vi "Process_single.vi"(0 "Arrays in":T2, 1 "output cluster":cluster{dbl, dbl, dbl, dbl}, 2 "Magnetic field":dbl, 3 "Calibration Constant (1/deg)":dbl) -> (5 "Magnetic_field_array":dbl[](array[numeric]), 6 "Time":dbl, 7 "Lockin_Y_array (V)":dbl[](array[numeric]), 8 "Time array (s)":dbl[](array[numeric]), 9 "Moke out":T1, 10 "LockIn Y":dbl, 11 "Lockin_R_array (V)":dbl[](array[numeric]), 12 "Lockin_Theta_array":dbl[](array[numeric]), 13 "LockIn R":dbl, 14 "LockIn X":dbl, 15 "MOKE_array (deg)":dbl[](array[numeric]), 16 "Lockin_X_array (V)":dbl[](array[numeric]), 17 "LockIn Theta":dbl, 18 "Dc_Voltage_array (V)":dbl[](array[numeric]))   [LabVIEW 2015]
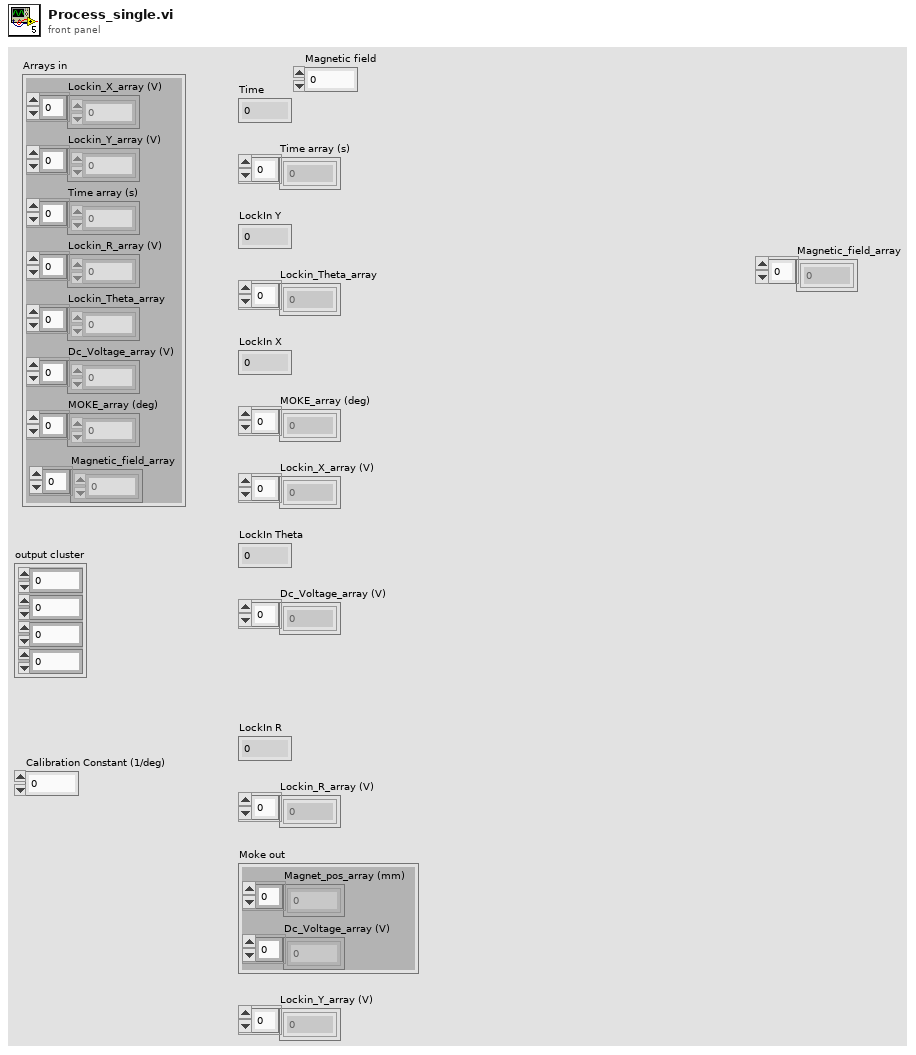
[diagram p1: front panel]
types:
  T1 = cluster{"Magnet_pos_array (mm)":dbl[], "Dc_Voltage_array (V)":dbl[]}
  T2 = cluster{"Lockin_X_array (V)":dbl[], "Lockin_Y_array (V)":dbl[], "Time array (s)":dbl[], "Lockin_R_array (V)":dbl[], "Lockin_Theta_array":dbl[], "Dc_Voltage_array (V)":dbl[], "MOKE_array (deg)":dbl[], "Magnetic_field_array":dbl[]}
  T3 = cluster{"Magnetic_field_array":dbl[], "Lockin_R_array (V)":dbl[]}
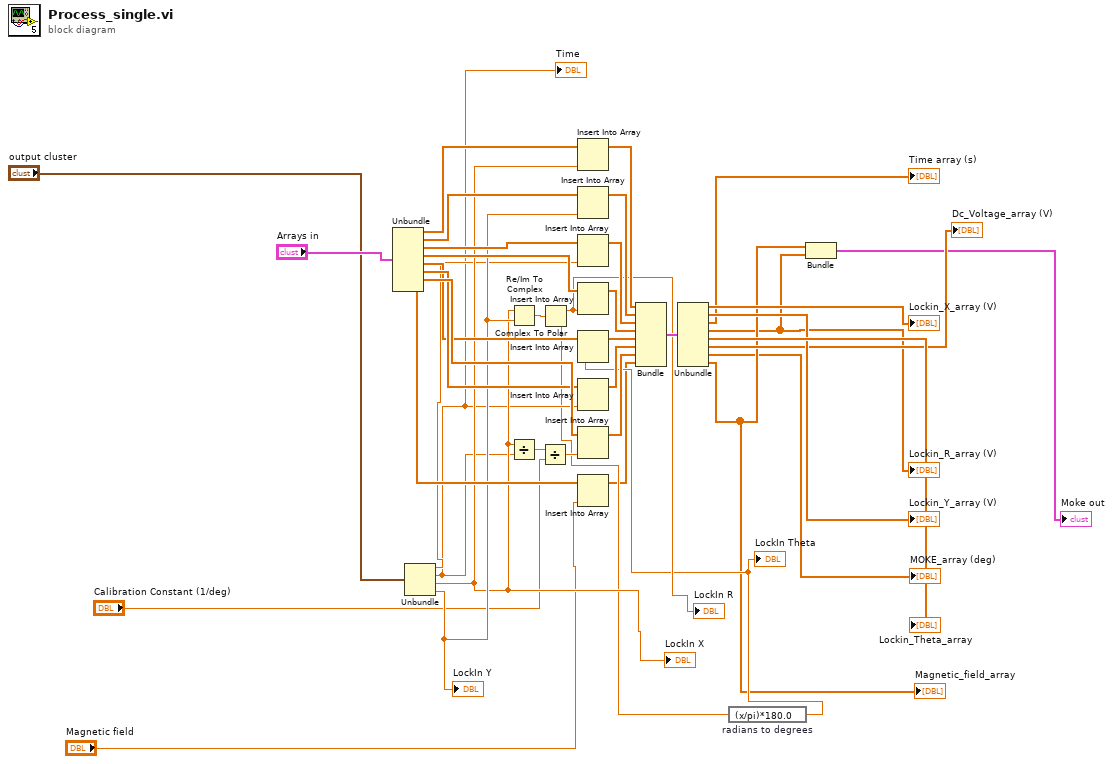
[diagram p0: block diagram]
diagram:
  n1 = Unbundle("Arrays in") -> ("Lockin_X_array (V)"=w22:dbl[], "Lockin_Y_array (V)"=w23:dbl[], "Time array (s)"=w24:dbl[], "Lockin_R_array (V)"=w25:dbl[], "Lockin_Theta_array"=w26:dbl[], "Dc_Voltage_array (V)"=w27:dbl[], "MOKE_array (deg)"=w28:dbl[], "Magnetic_field_array"=w29:dbl[])
  n2 = Unbundle("output cluster") -> (w16:dbl, w15:dbl, w17:dbl, w18:dbl)
  "LockIn Y" <- w18
  "LockIn X" <- w17
  "Time" <- w15
  n3 = Re/Im To Complex(1:w18, 2:w17) -> (0:w19:cdb)
  n4 = Divide(x=w17, y=w15) -> (x/y=w11:dbl)
  n5 = Divide(x=w11, y="Calibration Constant (1/deg)") -> (x/y=w13:dbl)
  n6 = Complex To Polar(r * e^(i*theta)=w19) -> (r=w20:dbl, theta=w10:dbl)
  "LockIn R" <- w20
  n7 = Insert Into Array(array=w22, new element=w17) -> (w32:dbl[])  [unwired: 1 in]
  n8 = Insert Into Array(array=w23, new element=w18) -> (w34:dbl[])  [unwired: 1 in]
  n9 = Insert Into Array(array=w24, new element=w16) -> (w31:dbl[])  [unwired: 1 in]
  n10 = Insert Into Array(array=w25, new element=w20) -> (w36:dbl[])  [unwired: 1 in]
  n11 = Insert Into Array(array=w27, new element=w15) -> (w39:dbl[])  [unwired: 1 in]
  n12 = Insert Into Array(array=w28, new element=w13) -> (w40:dbl[])  [unwired: 1 in]
  n13 = Insert Into Array(array=w29, new element="Magnetic field") -> (w6:dbl[])  [unwired: 1 in]
  n14 = expression code="(x/pi)*180.0" "radians to degrees"(w10) -> (w7:dbl)
  "LockIn Theta" <- w7
  n15 = Insert Into Array(array=w26, new element=w7) -> (w37:dbl[])  [unwired: 1 in]
  n16 = Bundle("Lockin_X_array (V)"=w32, "Lockin_Y_array (V)"=w34, "Time array (s)"=w31, "Lockin_R_array (V)"=w36, "Lockin_Theta_array"=w37, "Dc_Voltage_array (V)"=w39, "MOKE_array (deg)"=w40, "Magnetic_field_array"=w6) -> (w30:T2)  [unwired: 1 in]
  n17 = Unbundle(w30) -> ("Lockin_X_array (V)"=→"Lockin_X_array (V)":dbl[], "Lockin_Y_array (V)"=→"Lockin_Y_array (V)":dbl[], "Time array (s)"=→"Time array (s)":dbl[], "Lockin_R_array (V)"=w1:dbl[], "Lockin_Theta_array"=→"Lockin_Theta_array":dbl[], "Dc_Voltage_array (V)"=→"Dc_Voltage_array (V)":dbl[], "MOKE_array (deg)"=→"MOKE_array (deg)":dbl[], "Magnetic_field_array"=w4:dbl[])
  "Lockin_R_array (V)" <- w1
  "Magnetic_field_array" <- w4
  n18 = Bundle("Magnetic_field_array"=w4, "Lockin_R_array (V)"=w1) -> (→"Moke out":T3)  [unwired: 1 in]
